vi "Generate Signal.vi"(8 "error in (no error)":errorcluster, 11 "Signal Waveform in":refnum<class "Signal Waveform.lvclass">) -> (0 "error out":errorcluster, 3 "Signal Waveform out":refnum<class "Signal Waveform.lvclass">)   [LabVIEW 2020, in "Signal Waveform.lvclass"]
uses:
  Signal Waveform.lvclass
  Signal Waveform.lvclass/Signal Waveform.ctl
  <vilib>/measure/NI_MABase.lvlib
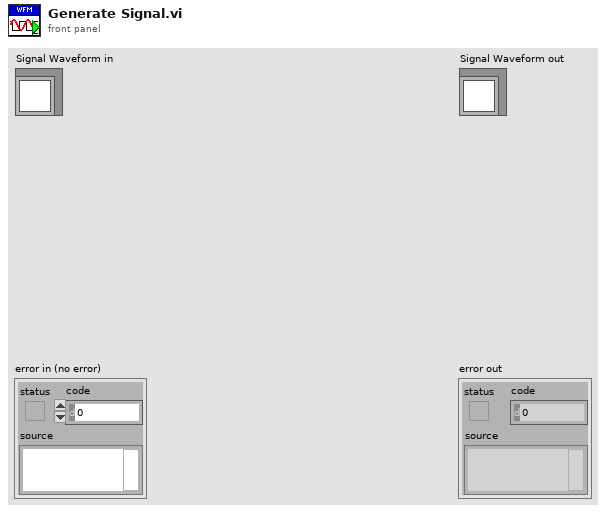
[diagram p1: front panel]
types:
  T1 = enum16{"Sine Wave", "Triangle Wave", "Square Wave", "Sawtooth Wave"}
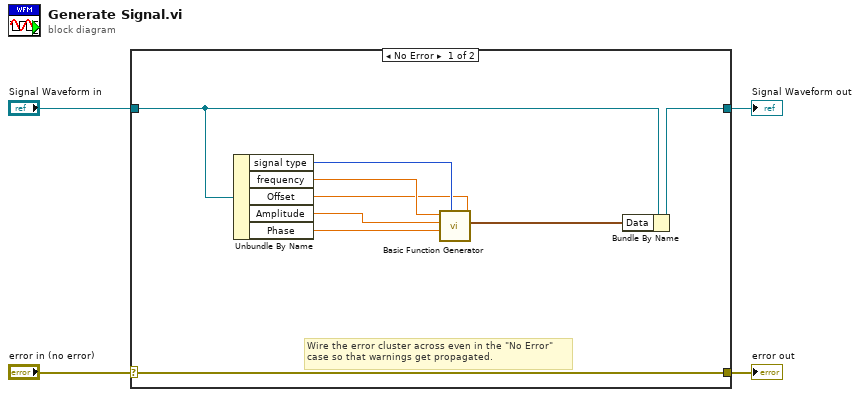
[diagram p0: block diagram]
diagram:
  n1 = case shown="No Error" "error in (no error)" {
    selector: "error in (no error)" -> [w13 w15]
    tunnel: [w13 w15] -> w3
    tunnel: [w10 w14] -> w1
    tunnel: "Signal Waveform in" -> [w12 w14]
    frame No Error {
      # "Wire the error cluster across even in the \"No Error\"\ncase so that warnings get propagated."
      n2 = Unbundle By Name(w12) -> ("signal type"=w8:T1, "frequency"=w11:dbl, "Offset"=w7:dbl, "Amplitude"=w5:dbl, "Phase"=w6:dbl)
      n3 = call <vilib>:"Basic Function Generator.vi"("offset"=w7, "signal type"=w8, "phase"=w6, "amplitude"=w5, "frequency"=w11) -> ("signal out"=w9:waveform(dbl))  [unwired: 4 in, 2 out]
      n4 = Bundle By Name(cluster=w12, "Data"=w9) -> (w10:refnum<class "Signal Waveform.lvclass">)
    }
    frame Error {
    }
  }
  "error out" <- w3
  "Signal Waveform out" <- w1
